vi "CS POLARIS BME DG Client.constructor.vi"(0 "name":string, 2 "data in":string, 5 "error in (no error)":errorcluster) -> (14 "i ref out":refnum<vi>, 16 "data out":string, 19 "error out":errorcluster)   [LabVIEW 2009, in "CS POLARIS BME DG Client.lvlib"]
doc: "This is the constructor of a class.\n\nLicense Agreement for this software:\n\nCopyright (C)\nGesellschaft für Schwerionenforschung, GSI\nPlanckstr. 1\n64291 Darmstadt\nGermany\n\nContact: D.Beck@gsi.de \n\nThis program is free software; you can redistribute it and/or modify it under the terms of the \nGNU General Public License as published by the Free Software Foundation; either version 2 of \nthe license, or (at your option) any later version.\n\nThis program is distributed in the hope that it will be useful, but WITHOUT ANY WARRANTY; \nwithout even the implied warranty of MERCHANTABILITY or FITNESS FOR A PARTICULAR PURPOSE. See the GNU General License for more details (http://www.gnu.org).\n\nGesellschaft für Schwerionenforschung, GSI\nPlanckstr. 1, 64291 Darmstadt, Germany\nFor all questions and ideas contact: M.Richter@gsi.de, H.Brand@gsi.de or D.Beck@gsi.de.\nLast update: 16-JUN-2004"
uses:
  CS POLARIS BME DG Client.lvlib
  CSCore/BaseProcess/BaseProcess.lvlib
  CSCore/CSSystem/CSSystemLib/CSSystemLib.lvlib
  CSCore/BaseGUI/BaseGUI.lvlib
  CSCore/CSObj/CSObj.lvlib
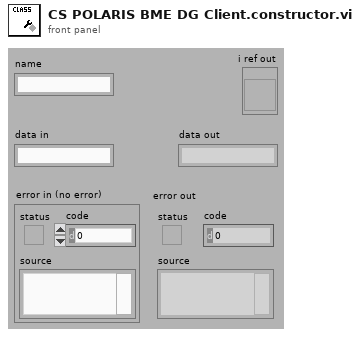
[diagram p1: front panel]
types:
  T1 = enum16{"SetAttribute", "GetAttribute", "CreateAttribute", "DestroyAttribute", "DestroyAllAtributes"}
  T2 = typedef "BaseProcess.lvlib/BaseProcess.i attribute.ctl" = cluster{"EventStatus":string, "EventError":i32, "PresetEvtWatchD":i32, "PresetPdcWatchD":i32, "EventTimeout":i32, "PeriodicInterval":i32, "Interface":string[], "Address":string[], "Special":string[], "PeriodicError":i32, "PeriodicStatus":string, "SuperProc":string, "Descriptors":T3[], "CaseRef":refnum<vi>, "PdcRef":refnum<vi>, "Thread Ref":refnum<vi>, "eventErrorID":i32, "eventStatusID":i32, "periodicErrorID":i32, "periodicStatusID":i32, "pdcCtrID":i32}
  T3 = typedef "BaseProcess.lvlib/BaseProcess.descriptor definition.ctl" = cluster{"selector":string, "descriptor":T4}
  T4 = typedef "BaseProcess.lvlib/BaseProcess.descriptor string definition.ctl" = string
  T5 = typedef "CS POLARIS BME DG Client.lvlib/CS POLARIS BME DG Client.i attribute.ctl" = cluster{"Delay Formula Ref":refnum<vi>, "Active Ref":refnum<vi>, "OutputModulo Ref":refnum<vi>, "Rep Rate Ref":refnum<vi>, "Next Shot Ref":refnum<vi>, "Error Ref":refnum<vi>, "Switch Ref":refnum<vi>, "New Delay Formula Ref":refnum<vi>, "New OutputModulo Ref ":refnum<vi>, "Channel":string, "CS DG Obj":string, "Stop Ref":refnum<vi>}
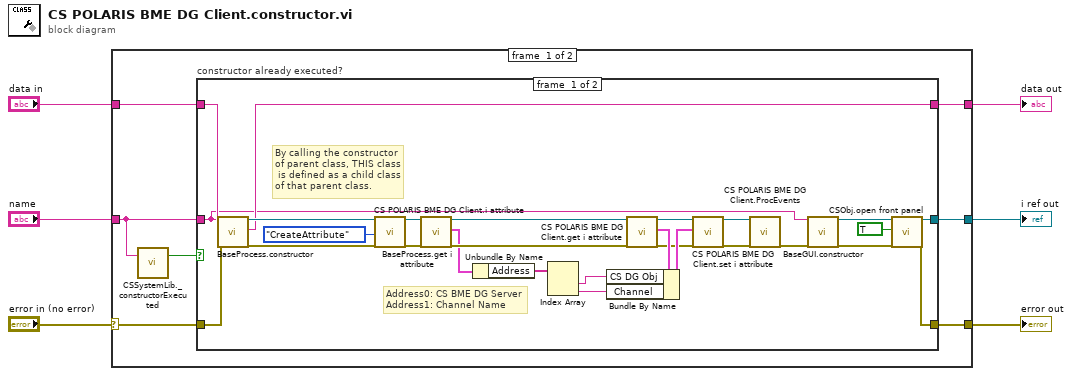
[diagram p0: block diagram]
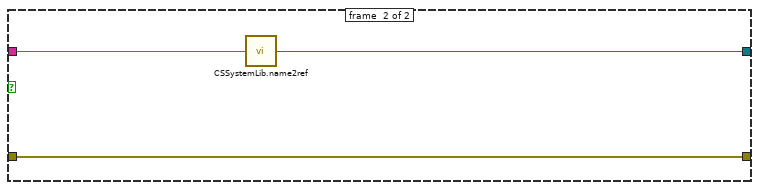
[diagram p2: hidden frame]
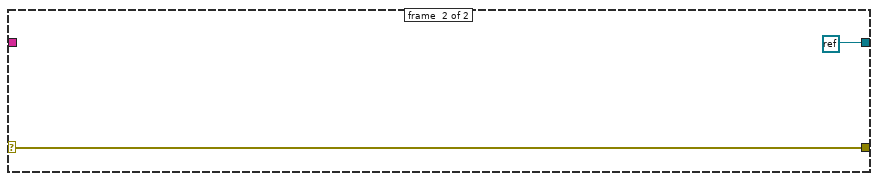
[diagram p3: hidden frame]
diagram:
  n1 = case shown="No Error" "error in (no error)" {
    selector: "error in (no error)" -> [w11 w44]
    tunnel: "name" -> [w10 _]
    tunnel: [w13 refnum<k0> refnum] -> w5
    tunnel: [w12 w44] -> w4
    tunnel: "data in" -> [w8 _]
    tunnel: [w7 _] -> w1
    frame #0 {
      n2 = call "CSSystemLib._constructorExecuted.vi"("name"=w10) -> ("constructor executed?"=w9:bool)  [unwired: 18 in]
      n3 = case "constructor already executed?" shown="False" w9 {
        tunnel: [w31 w42] -> w13
        tunnel: [w29 w41] -> w12
        tunnel: w11 -> [w37 w41]
        tunnel: w10 -> [w33 w43]
        tunnel: w8 -> [w36 _]
        tunnel: [w35 _] -> w7
        frame #0 {
          # "Address0: CS BME DG Server\nAddress1: Channel Name"
          # "By calling the constructor\nof parent class, THIS class\n is defined as a child class\nof that parent class."
          n4 = call "BaseProcess.constructor.vi"("name"=w33, "data in"=w36, "error in (no error)"=w37) -> ("i ref out"=w40:refnum<vi>, "data out"=w35:string, "error out"=w39:errorcluster)  [unwired: 14 in]
          n5 = call "CS POLARIS BME DG Client.i attribute.vi"("VI Refnum"=w40, "Action"=T1."CreateAttribute", "error in (no error)"=w39) -> ("VI Refnum out"=w19:refnum<vi>, "error out"=w27:errorcluster)  [unwired: 14 in, 1 out]
          n6 = call "BaseProcess.get i attribute.vi"("i ref in"=w19, "error in (no error)"=w27) -> ("i ref out"=w18:refnum<vi>, "i attribute"=w17:T2, "error out"=w20:errorcluster)  [unwired: 15 in]
          n7 = Unbundle By Name(w17) -> ("Address"=w16:string[])
          n8 = Index Array(array=w16) -> (element #1=w15:string, element #2=w14:string)  [unwired: 2 in]
          n9 = call "CS POLARIS BME DG Client.get i attribute.vi"("i ref in"=w18, "error in (no error)"=w20) -> ("i ref out"=w26:refnum<vi>, "i attribute"=w25:T5, "error out"=w21:errorcluster)  [unwired: 15 in]
          n10 = Bundle By Name(cluster=w25, "CS DG Obj"=w15, "Channel"=w14) -> (w24:T5)
          n11 = call "CS POLARIS BME DG Client.set i attribute.vi"("i ref in"=w26, "i attribute"=w24, "error in (no error)"=w21) -> ("i ref out"=w23:refnum<vi>, "error out"=w22:errorcluster)  [unwired: 15 in]
          n12 = call "CS POLARIS BME DG Client.ProcEvents.vi"("i ref in"=w23, "error in (no error)"=w22) -> ("error out"=w34:errorcluster)  [unwired: 16 in, 1 out]
          n13 = call "BaseGUI.constructor.vi"("name"=w33, "error in (no error)"=w34) -> ("i ref out"=w32:refnum<vi>, "error out"=w30:errorcluster)  [unwired: 15 in, 1 out]
          n14 = call "CSObj.open front panel.vi"("i ref in"=w32, "frontPanelOpen"=TRUE, "error in (no error)"=w30) -> ("i ref out"=w31:refnum<vi>, "error out"=w29:errorcluster)  [unwired: 15 in]
        }
        frame #1 {
          n15 = call "CSSystemLib.name2ref.vi"("name"=w43) -> ("obj refnum"=w42:refnum<vi>)
        }
      }
    }
    frame #1 {
    }
  }
  "i ref out" <- w5
  "error out" <- w4
  "data out" <- w1
